vi "Parse Setup file.vi"(0 "Data In":string[][](array[string])) -> (3 "IP Address":string, 4 "Environment Details":string[][](array[string]), 6 "Instrument Identification":string[][](array[string]), 8 "Calibration Details":string[][](array[string]), 10 "Standards Used":string[][](array[string]), 14 "Channel Descriptions w/ Tracking":string[][](array[string]), 15 "Machine Specifications":string[][](array[string]))   [LabVIEW 2013]
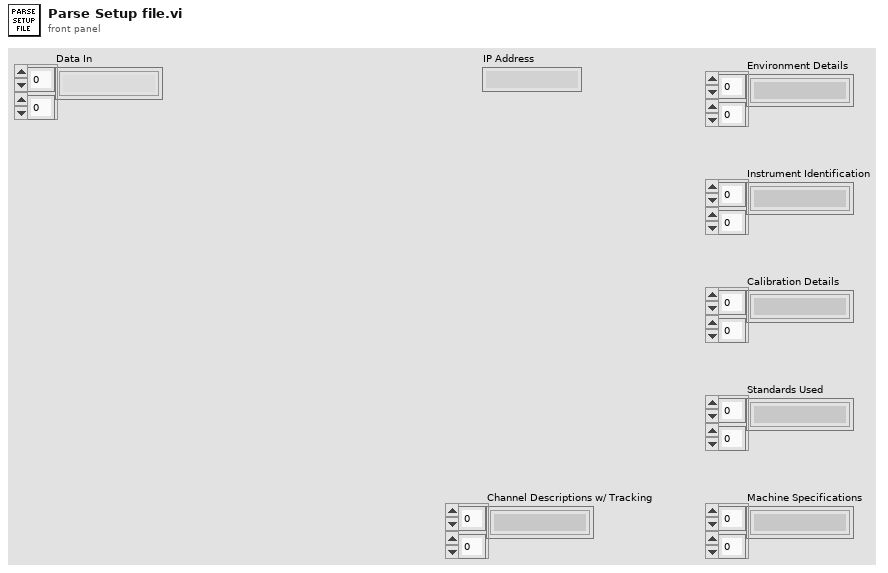
[diagram p1: front panel]
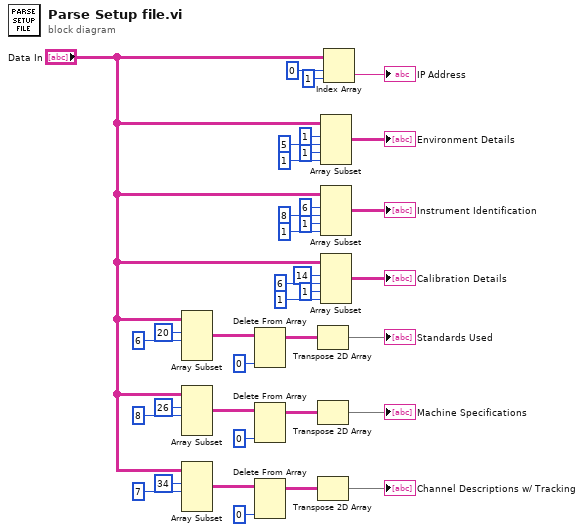
[diagram p0: block diagram]
diagram:
  n1 = Array Subset(array="Data In", index (row)=20 ("index"), length (row)=6 ("length")) -> (w17:string[][])  [unwired: 2 in]
  n2 = Array Subset(array="Data In", index (row)=26 ("index"), length (row)=8 ("length")) -> (w12:string[][])  [unwired: 2 in]
  n3 = Array Subset(array="Data In", index (row)=34 ("index"), length (row)=7 ("length")) -> (w5:string[][])  [unwired: 2 in]
  n4 = Delete From Array(array=w17, index (col)=0 ("disabled index (col)")) -> (array with subset deleted=w15:string[][])  [unwired: 2 in, 1 out]
  n5 = Delete From Array(array=w12, index (col)=0 ("disabled index (col)")) -> (array with subset deleted=w14:string[][])  [unwired: 2 in, 1 out]
  n6 = Delete From Array(array=w5, index (col)=0 ("disabled index (col)")) -> (array with subset deleted=w3:string[][])  [unwired: 2 in, 1 out]
  n7 = Transpose 2D Array(2D array=w15) -> (transposed array=→"Standards Used":string[][])
  n8 = Transpose 2D Array(2D array=w14) -> (transposed array=→"Machine Specifications":string[][])
  n9 = Transpose 2D Array(2D array=w3) -> (transposed array=→"Channel Descriptions w/ Tracking":string[][])
  n10 = Array Subset(array="Data In", index (row)=1 ("index"), length (row)=5 ("length"), index (col)=1 ("index"), length (col)=1 ("length")) -> (→"Environment Details":string[][])
  n11 = Array Subset(array="Data In", index (row)=6 ("index"), length (row)=8 ("length"), index (col)=1 ("index"), length (col)=1 ("length")) -> (→"Instrument Identification":string[][])
  n12 = Array Subset(array="Data In", index (row)=14 ("index"), length (row)=6 ("length"), index (col)=1 ("index"), length (col)=1 ("length")) -> (→"Calibration Details":string[][])
  n13 = Index Array(array="Data In", index (row)=0 ("disabled index (row)"), index (col)=1 ("disabled index (col)")) -> (element=→"IP Address":string)
